vi "pp2_DAQstopAudio.vi"(0 "Daq config In":T1={"Sound AO"="Dev2/ao0", "Shock intesity AO"="Dev1/ao1", "Code_LED DO"="Dev1/port1:2", "Switch DI"="Dev1/port0/line0:1", "Webcam"="cam0", "Sound AO task"="", "Sound card task"=0, "Shock intensity AO task"="", "Code_LED DO task"="", "Switch DI task"="", "AO <=> Sound card"=FALSE, "Sound card"=0, "sample rate"=8000.0, "Variable shock"=FALSE, "Webcam on"=FALSE, "Tone gate PFI"="/Dev1/PFI1", "Waveform memo"={"t0"=timestamp(0 s since 1904-01-01), "dt"=1.0, "Y"=[]}, "First time"=FALSE} {"sample rate" min=8000.0; "Sound card task" format="%.0x"}, 11 "error in (no error)":errorcluster) -> (4 "Daq config Out":T1={"Sound AO"="Dev2/ao0", "Shock intesity AO"="Dev1/ao1", "Code_LED DO"="Dev1/port1:2", "Switch DI"="Dev1/port0/line0:1", "Webcam"="cam0", "Sound AO task"="", "Sound card task"=0, "Shock intensity AO task"="", "Code_LED DO task"="", "Switch DI task"="", "AO <=> Sound card"=FALSE, "Sound card"=0, "sample rate"=8000.0, "Variable shock"=FALSE, "Webcam on"=FALSE, "Tone gate PFI"="/Dev1/PFI1", "Waveform memo"={"t0"=timestamp(0 s since 1904-01-01), "dt"=1.0, "Y"=[]}, "First time"=FALSE} {"sample rate" min=8000.0; "Sound card task" format="%.0x"}, 15 "error out":errorcluster)   [LabVIEW 2013]
uses:
  pp2_CTL_DaqConfig.ctl
  <vilib>/userdefined/High Color/IMAQdx.ctl
  <vilib>/sound2/lvsound2.llb/Sound Output Task ID.ctl
  <resource>/objmgr/daqmx.rc
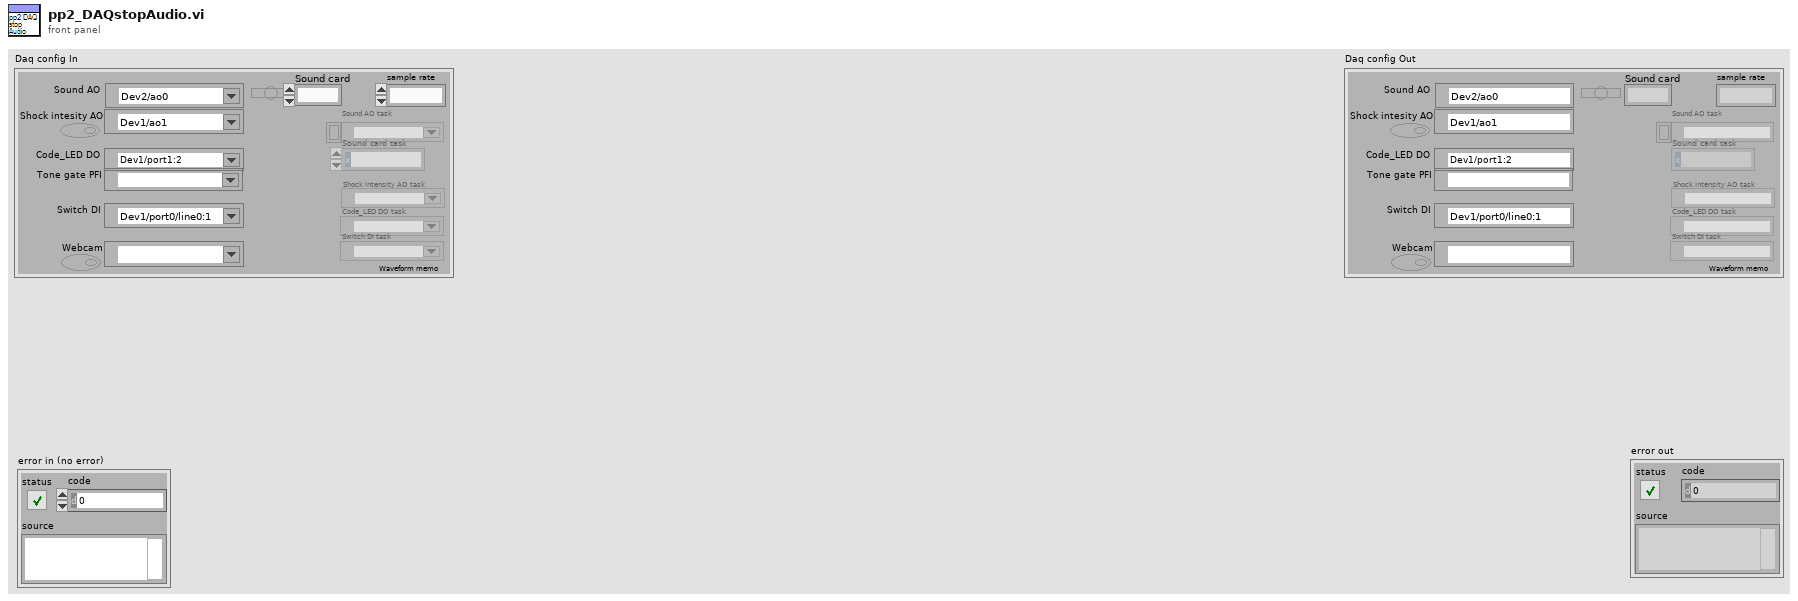
[diagram p1: front panel]
types:
  T1 = typedef "pp2_CTL_DaqConfig.ctl" = cluster{"Sound AO":tag, "Shock intesity AO":tag, "Code_LED DO":tag, "Switch DI":tag, "Webcam":T2, "Sound AO task":refnum<k21>, "Sound card task":T3, "Shock intensity AO task":refnum<k21>, "Code_LED DO task":refnum<k21>, "Switch DI task":refnum<k21>, "AO <=> Sound card":bool, "Sound card":u32, "sample rate":dbl, "Variable shock":bool, "Webcam on":bool, "Tone gate PFI":tag, "Waveform memo":waveform(dbl), "First time":bool}
  T2 = typedef "IMAQdx.ctl" = refnum<k21>
  T3 = typedef "Sound Output Task ID.ctl" = u32
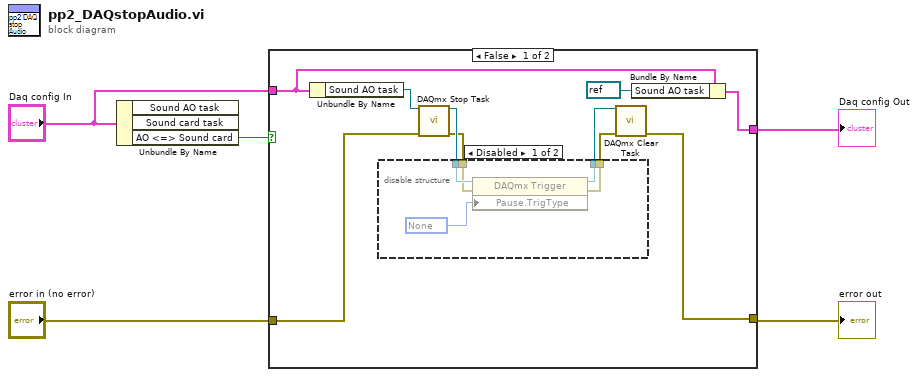
[diagram p0: block diagram]
diagram:
  n1 = Unbundle By Name("Daq config In") -> ("AO <=> Sound card"=w3:bool)  [unwired: 2 out]
  n2 = case shown="False" w3 {
    tunnel: "error in (no error)" -> [w15 w24]
    tunnel: [w14 w24] -> w4
    tunnel: "Daq config In" -> [w12 w23]
    tunnel: [w13 w23] -> w1
    frame False {
      n3 = Unbundle By Name(w12) -> ("Sound AO task"=w11:refnum<k21>)
      n4 = call <vilib>:"DAQmx Stop Task.vi"("task/channels in"=w11, "error in"=w15) -> ("task out"=w9:refnum<k21>, "error out"=w8:errorcluster)  [unwired: 12 in]
      n5 = disable-structure shown="Disabled" {
        disable-tunnel: w9 -> [w20 w22]
        disable-tunnel: w8 -> [w19 w21]
        disable-tunnel: [w18 w22] -> w7
        disable-tunnel: [w17 w21] -> w6
        frame Disabled {
          w16 = 10230 items=["Analog Level"=10101, "Analog Window"=10103, "Digital Level"=10152, "Digital Pattern"=10398, "None"=10230] ("Pause.TrigType")
          n6 = property class="DAQmx Trigger"(reference=w20, error in=w19, "Pause.TrigType"=w16) -> (reference out=w18:refnum<k21>, error out=w17:errorcluster)
        }
        frame Enabled {
        }
      }
      n7 = call <vilib>:"DAQmx Clear Task.vi"("task in"=w7, "error in"=w6) -> ("error out"=w14:errorcluster)  [unwired: 13 in]
      n8 = Bundle By Name(cluster=w12, "Sound AO task"=refnum<k21> refnum) -> (w13:T1)
    }
    frame True {
    }
  }
  "Daq config Out" <- w1
  "error out" <- w4
